vi "Gasteiler abgleichen.vi"(10 "Gasteiler":T1, 11 "Gasteilerliste":T1) -> (3 "x != y?":bool)   [LabVIEW 2020, in "System Einstellungen V2.lvlib"]
uses:
  System Einstellungen V2.lvlib
  <vilib>/Utility/miscctls.llb/LVStringsAndValuesArrayTypeDef.ctl
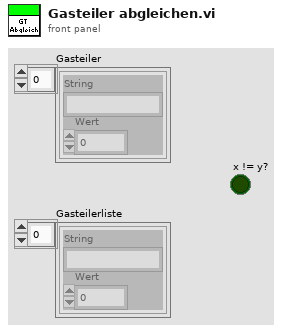
[diagram p1: front panel]
types:
  T1 = typedef "LVStringsAndValuesArrayTypeDef.ctl" = cluster{"String":string, "Value":ext}[]
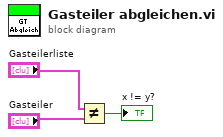
[diagram p0: block diagram]
diagram:
  n1 = Not Equal?(x="Gasteilerliste", y="Gasteiler") -> (x != y?=→"x != y?":bool)
